vi "RSZVB Set Local Oscilator A State.vi"(7 "State (T: On)":bool=TRUE, 8 "error in (no error)":errorcluster {"code" format="%.0x"}, 9 "Port (1)":i32=1, 10 "Channel (1)":i32=1, 11 "VISA session":refnum<visa-resource-name>) -> (0 "error out":errorcluster {"code" format="%.0x"}, 3 "dup VISA session":refnum<visa-resource-name>)   [LabVIEW 2011]
doc: "This VI switches the Local Oscillator amplifier for the reference channel a on or off. \n\nRemote-control command(s):\n[SENSe<Ch>:]LOReference<Pt>[:STATe] <Boolean>"
uses:
  _utility/RSZVB Global Data.vi
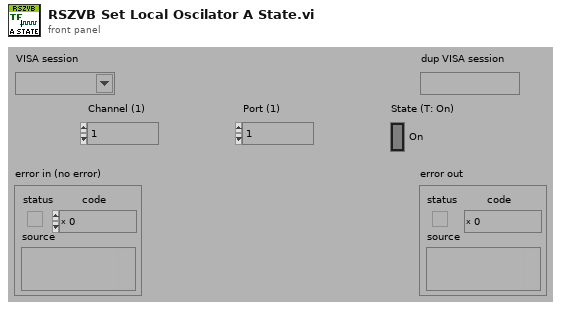
[diagram p1: front panel]
types:
  T1 = cluster{"Error Checking (T: On)":bool, "Installed Options":string[], "Data Valid?":bool, "Ports":i32, "Model":string[], "Option Checking (T: On)":bool}[]
  T2 = cluster{"Error Checking (T: On)":bool, "Installed Options":string[], "Data Valid?":bool, "Ports":i32, "Model":string[], "Option Checking (T: On)":bool}
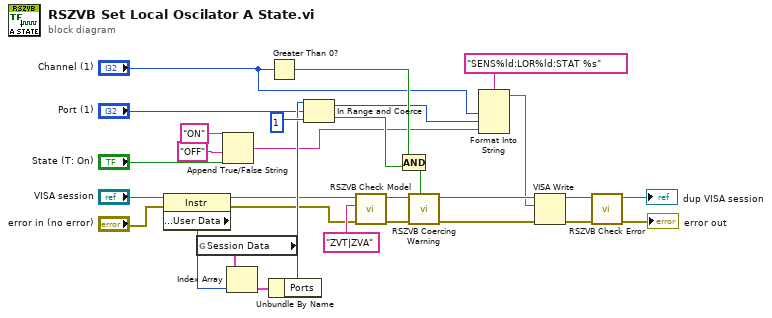
[diagram p0: block diagram]
diagram:
  n1 = property class="Instr"(reference="VISA session", error in="error in (no error)") -> (reference out=w2:refnum<visa-resource-name>, error out=w1:errorcluster, "General Settings:User Data"=w19:u32)
  n2 = global read "RSZVB Global Data.vi" "Session Data"() -> (w20:T1)
  n3 = Append True/False String(1:"State (T: On)", 2:"OFF", 3:"ON") -> (0:w6:string)  [unwired: 1 in]
  n4 = Index Array(array=w20, index=w19) -> (element=w21:T2)
  n5 = Greater Than 0?(x="Channel (1)") -> (x > 0?=w22:bool)
  n6 = Unbundle By Name(w21) -> ("Ports"=w13:i32)
  n7 = In Range and Coerce(upper limit=w13, x="Port (1)", lower limit=1) -> (coerced(x)=w7:i32, In Range?=w11:bool)
  n8 = call "RSZVB Check Model.vi"("error in (no error)"=w1, "Model"="ZVT|ZVA" ("Options"), "VISA session"=w2) -> ("error out"=w4:errorcluster, "dup VISA session"=w3:refnum<visa-resource-name>)  [unwired: 7 in]
  n9 = Compound Arithmetic op=AND(w22, w11) -> (w24:bool)
  n10 = call "RSZVB Coercing Warning.vi"("In Range?"=w24, "error in (no error)"=w4, "VISA session"=w3) -> ("error out"=w27:errorcluster, "dup VISA session"=w28:refnum<visa-resource-name>)  [unwired: 7 in]
  n11 = Format Into String(format string="SENS%ld:LOR%ld:STAT %s", "Channel (1)", w7, w6) -> (resulting string=w23:string)  [unwired: 2 in, 1 out]
  n12 = VISA Write(VISA resource name=w28, write buffer=w23, error in (no error)=w27) -> (VISA resource name out=w25:refnum<visa-resource-name>, error out=w26:errorcluster)  [unwired: 1 out]
  n13 = call "RSZVB Check Error.vi"("error in (no error)"=w26, "VISA session"=w25) -> ("error out"=→"error out":errorcluster, "dup VISA session"=→"dup VISA session":refnum<visa-resource-name>)  [unwired: 8 in]
